vi "setImageRefGray.vi"(8 "error in (no error)":errorcluster, 10 "Image":T1, 11 "camera in":refnum<class "camera.lvclass">) -> (0 "error out":errorcluster, 3 "camera out":refnum<class "camera.lvclass">)   [LabVIEW 2017, in "camera.lvclass"]
uses:
  camera.lvclass
  <vilib>/vision/Image Controls.llb/IMAQ Image.ctl
  camera.lvclass/camera.ctl
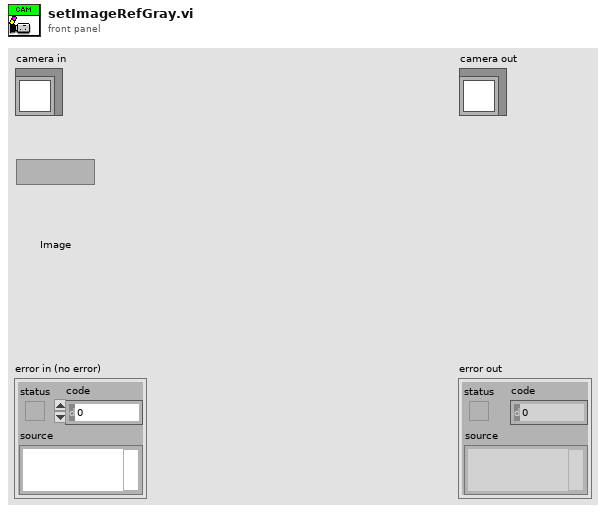
[diagram p1: front panel]
types:
  T1 = typedef "IMAQ Image.ctl" = refnum<image>
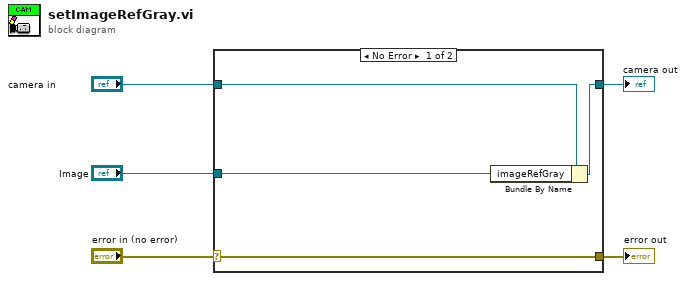
[diagram p0: block diagram]
diagram:
  n1 = case shown="No Error" "error in (no error)" {
    selector: "error in (no error)" -> [w9 w10]
    tunnel: [w9 w10] -> w4
    tunnel: [w7 w11] -> w2
    tunnel: "camera in" -> [w8 w11]
    tunnel: "Image" -> [w6 _]
    frame No Error {
      n2 = Bundle By Name(cluster=w8, "imageRefGray"=w6) -> (w7:refnum<class "camera.lvclass">)
    }
    frame Error {
    }
  }
  "error out" <- w4
  "camera out" <- w2
